vi "write_lockin_FP_DSC.vi"(8 "error in (no error)":errorcluster, 11 "front panel":T1={"AO Configuration"=[], "AI Configuration"=[], "Channels: AO"=[], "Channels: Lockin"=[{"Enable?"=FALSE, "Channel"=13, "Frequency"=0.1, "Phase"=0.0, "TC"=1e-05, "Roll-Off"=1}], "DAQ Type"=enum."None", "Amplifiers"=enum."Manual", "Gain"=[], "offsets"=[], "Cal Info"=[], "TC (s)"=0.0, "order"=0, "60 Hz prefilter"=FALSE, "LP prefilter"=FALSE, "LP cutoff (Hz)"=0.0, "Fs"=0, "#s"=0} {"AI Configuration"."AI.Coupling" items=["AC"=10045, "DC"=10050, "GND"=10066]; "Channels: AO"."Phase" format="%.3g"; "Channels: AO"."Frequency" min=0.0001 max=10000.0 format="%.3g"; "Channels: AO"."Offset" format="%.3p"; "Channels: AO"."Amplitude" min=0.0 max=10.0 format="%.3p"; "Channels: Lockin"."Roll-Off" min=1; "Channels: Lockin"."TC" min=0.0001 format="%#_3p"; "Channels: Lockin"."Phase" format="%.3g"; "Channels: Lockin"."Frequency" min=0.0001 max=10000.0 format="%.3g"; "Cal Info"."SelfCal.LastDate/Time" format="%<%I:%M %p\n%m/%d/%Y>T"}) -> (0 "error out":errorcluster)   [LabVIEW 2019, in "Instrument.DAQ.lvclass"]
uses:
  Instrument.DAQ.lvclass
  <vilib>/addons/_JKI.lib/Serialization/JSON/JKI JSON Serialization.lvlib
  <vilib>/Utility/sysdir.llb/System Directory Type.ctl
  Typedefs/AmplifierType-enum.ctl
  Typedefs/DAQType-enum.ctl
  Typedefs/REF-cluster.ctl
  Typedefs/Function-enum.ctl
  Typedefs/AO-cluster.ctl
  Typedefs/AI.coupling-enum.ctl
  Typedefs/446xAI-enum.ctl
  Typedefs/AI.config(UI)-cluster.ctl
  Typedefs/AI.config(UI)-array.ctl
  Typedefs/446xAO-enum.ctl
  Typedefs/AO.config(UI)-cluster.ctl
  Typedefs/AO.config(UI)-array.ctl
  Typedefs/Front Panel Cluster.ctl
  Typedefs/Cal Info - Cluster.ctl
  Instrument UI.Lockin/Typedefs/REF Channel--Cluster.ctl
  Instrument UI.Lockin/Instrument UI.Lockin.lvclass
  Instrument UI.Lockin/Typedefs/AO Channel--Cluster.ctl
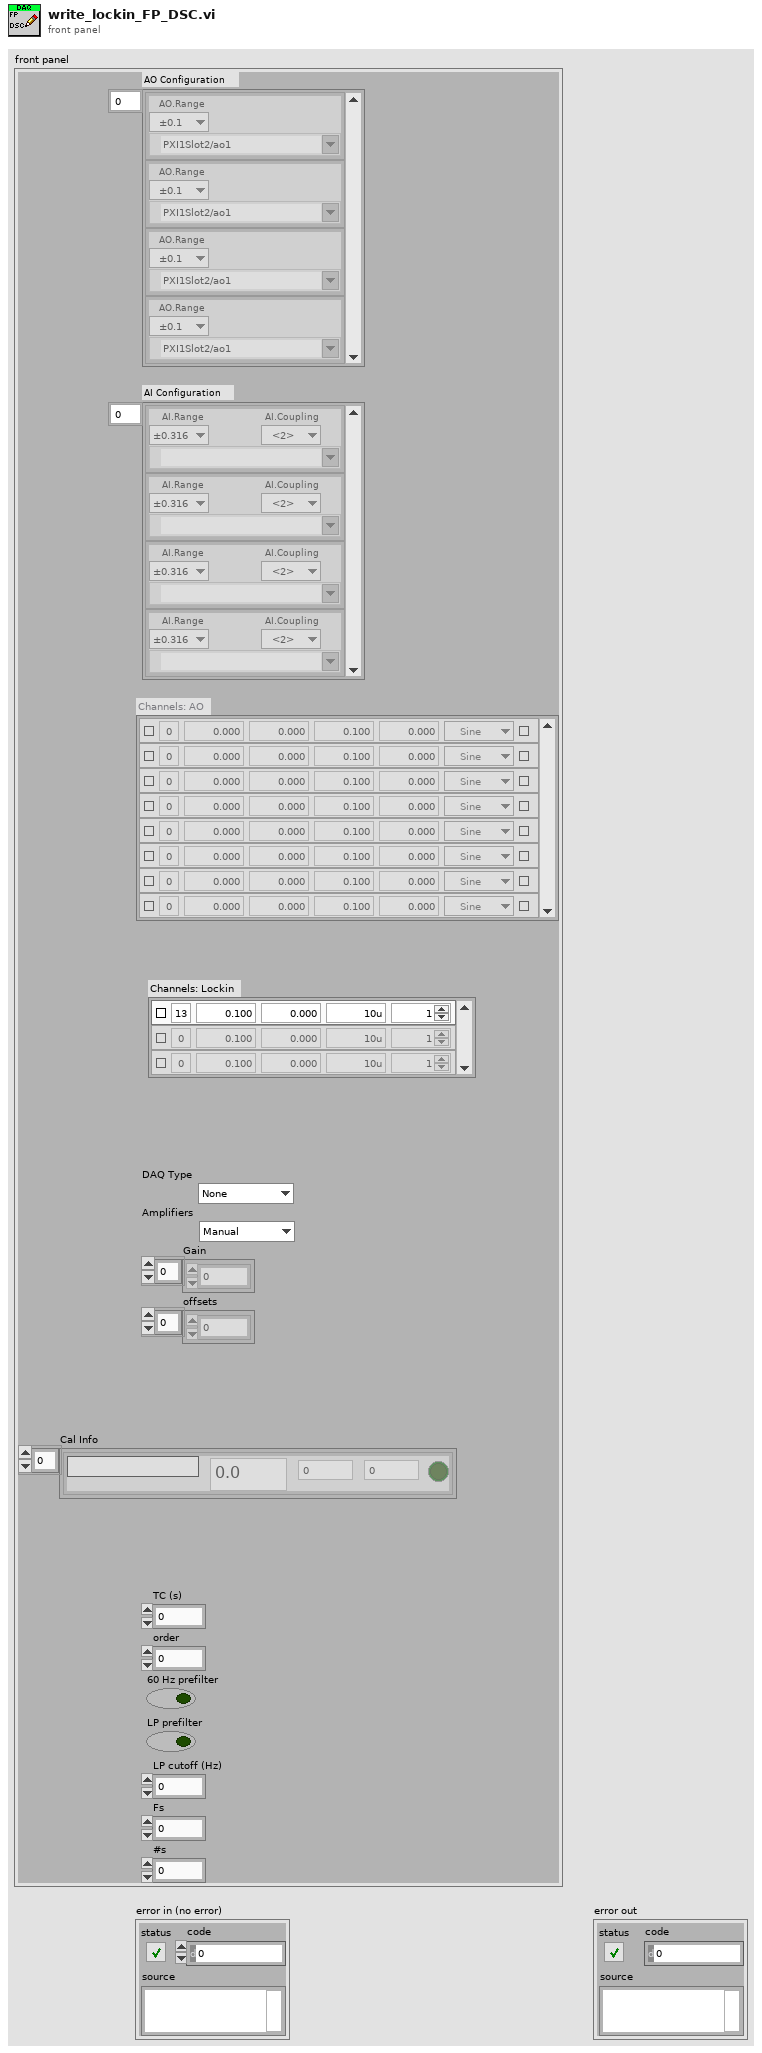
[diagram p1: front panel]
types:
  T1 = typedef "Instrument.DAQ.lvclass/Front Panel Cluster.ctl" = cluster{"AO Configuration":T2, "AI Configuration":T5, "Channels: AO":T9, "Channels: Lockin":T12, "DAQ Type":T14, "Amplifiers":T15, "Gain":dbl[], "offsets":dbl[], "Cal Info":T16[], "TC (s)":dbl, "order":i32, "60 Hz prefilter":bool, "LP prefilter":bool, "LP cutoff (Hz)":dbl, "Fs":i32, "#s":i32}
  T2 = typedef "Instrument.DAQ.lvclass/AO.config(UI)-array.ctl" = T3[]
  T3 = typedef "Instrument.DAQ.lvclass/AO.config(UI)-cluster.ctl" = cluster{"AO.Range":T4, "AO.channels":tag}
  T4 = typedef "Instrument.DAQ.lvclass/446xAO-enum.ctl" = enum16{"±0.1", "±1.0", "±10.0"}
  T5 = typedef "Instrument.DAQ.lvclass/AI.config(UI)-array.ctl" = T6[]
  T6 = typedef "Instrument.DAQ.lvclass/AI.config(UI)-cluster.ctl" = cluster{"AI.Coupling":T7, "AI.channels":tag, "AI.Range":T8}
  T7 = typedef "Instrument.DAQ.lvclass/AI.coupling-enum.ctl" = u16
  T8 = typedef "Instrument.DAQ.lvclass/446xAI-enum.ctl" = enum16{"±0.316", "±1.00", "±3.16", "±10.0", "±31.6", "±42.4"}
  T9 = typedef "Instrument.DAQ.lvclass/AO-cluster.ctl" = T10[]
  T10 = typedef "Instrument UI.Lockin.lvclass/AO Channel--Cluster.ctl" = cluster{"Enable?":bool, "Channel":i32, "Amplitude":dbl, "Offset":dbl, "Frequency":dbl, "Phase":dbl, "Function":T11, "Sweeping?":bool}
  T11 = typedef "Instrument.DAQ.lvclass/Function-enum.ctl" = enum16{"Sine", "Triangle", "Square"}
  T12 = typedef "Instrument.DAQ.lvclass/REF-cluster.ctl" = T13[]
  T13 = typedef "Instrument UI.Lockin.lvclass/REF Channel--Cluster.ctl" = cluster{"Enable?":bool, "Channel":i32, "Frequency":dbl, "Phase":dbl, "TC":dbl, "Roll-Off":i32}
  T14 = typedef "Instrument.DAQ.lvclass/DAQType-enum.ctl" = enum16{"None", "USB 4431", "PXI 446x"}
  T15 = typedef "Instrument.DAQ.lvclass/AmplifierType-enum.ctl" = enum16{"Manual", "Krohn Hite", "Femto"}
  T16 = typedef "Instrument.DAQ.lvclass/Cal Info - Cluster.ctl" = cluster{"Active Device":string, "SelfCal.LastDate/Time":dbl, "SelfCal.LastTemp":dbl, "DevTemp":dbl, "calibration due?":bool}
  T17 = typedef "System Directory Type.ctl" = i32
  T18 = cluster{"AO Configuration":cluster{"AO.Range":T4, "AO.channels":string}[], "AI Configuration":cluster{"AI.Coupling":T7, "AI.channels":string, "AI.Range":T8}[], "Channels: AO":T9, "Channels: Lockin":T12, "DAQ Type":T14, "Amplifiers":T15, "Gain":dbl[], "offsets":dbl[], "Cal Info":cluster{"Active Device":string, "SelfCal.LastDate/Time":timestamp, "SelfCal.LastTemp":dbl, "DevTemp":dbl, "calibration due?":bool}[], "TC (s)":dbl, "order":i32, "60 Hz prefilter":bool, "LP prefilter":bool, "LP cutoff (Hz)":dbl, "Fs":i32, "#s":i32}
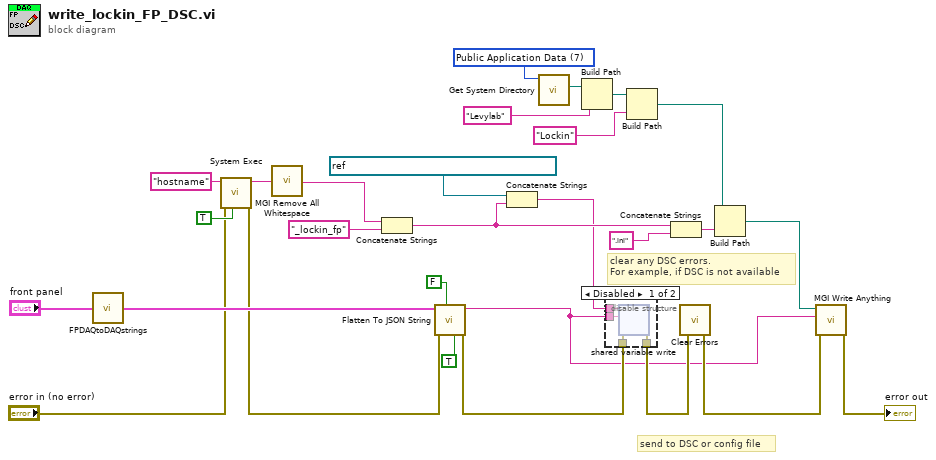
[diagram p0: block diagram]
diagram:
  w3 = T17 7 items=["User Home"=0, "User Desktop"=1, "User Documents"=2, "User Application Data"=3, "User Preferences"=4, "User Temporary"=5, "Public Documents"=6, "Public Application Data"=7, "Public Preferences"=8, "Public Cache"=13, "System Core Libraries"=9, "System Installed Libraries"=10, "Application Files"=11, "Boot Volume Root"=12] ("system directory type")
  # "clear any DSC errors.\nFor example, if DSC is not available"
  # "send to DSC or config file"
  n1 = call "FPDAQtoDAQstrings.vi"("front panel"="front panel") -> ("front panel (DAQmx strings)"=w23:T18)
  n2 = call <vilib>:"System Exec.vi"("run minimized? (F)"=TRUE, "error in (no error)"="error in (no error)", "command line"="hostname") -> ("error out"=w13:errorcluster, "standard output"=w16:string)  [unwired: 5 in, 2 out]
  n3 = call <userlib>:"MGI Remove All Whitespace.vi"("String"=w16) -> ("Trimmed String"=w11:string)
  n4 = Concatenate Strings(w11, "_lockin_fp" ("regular expression")) -> (w10:string)
  n5 = call <vilib>:"Flatten To JSON String.vi"("Enums As String (F)"=TRUE, "Multiline (T)"=FALSE, "error in (no error)"=w13, "Variant"=w23) -> ("error out"=w27:errorcluster, "JSON String"=w8:string)  [unwired: 6 in]
  n6 = Concatenate Strings(refnum<k21> "ni.var.psp://housesoftheholy/lockins/" ("shared variable refnum in"), w10) -> (w7:string)
  n7 = call <vilib>:"Get System Directory.vi"("system directory type"=w3) -> ("system directory"=w6:path)  [unwired: 10 in]
  n8 = Build Path(base path=w6, name or relative path="Levylab") -> (appended path=w4:path)
  n9 = disable-structure shown="Disabled" {
    disable-tunnel: w27 -> [w32 _]
    disable-tunnel: [w31 _] -> w22
    disable-tunnel: w8 -> [w30 _]
    disable-tunnel: w7 -> [w29 _]
    frame Disabled {
      n10 = shared-variable-write(w29, w32, w30) -> (w31:errorcluster)  [unwired: 1 out]
    }
    frame Enabled {
    }
  }
  n11 = Build Path(base path=w4, name or relative path="Lockin") -> (appended path=w1:path)
  n12 = Concatenate Strings(w10, ".ini" ("name or relative path")) -> (w19:string)
  n13 = call <vilib>:"Clear Errors.vi"("error in (no error)"=w22) -> ("error out"=w15:errorcluster)  [unwired: 5 in, 1 out]
  n14 = Build Path(base path=w1, name or relative path=w19) -> (appended path=w21:path)
  n15 = call <userlib>:"MGI Write Anything.vi"("Error In"=w15, "Anything"=w8, "Path (dialog)"=w21) -> ("Error Out"=→"error out":errorcluster)  [unwired: 6 in, 2 out]
